vi "Transition State.vi"(8 "Error In":errorcluster, 10 "L       E \nIndicator":T1 caption="L      E", 11 "Present  State":T2) -> (0 "Error Out":errorcluster, 3 "Next State":T2)   [LabVIEW 2023]
doc: "This VI uses the present state and thre inputs L and E to determine the next state."
uses:
  controls/enum defining states.ctl
  controls/Boolean L E indictaor.ctl
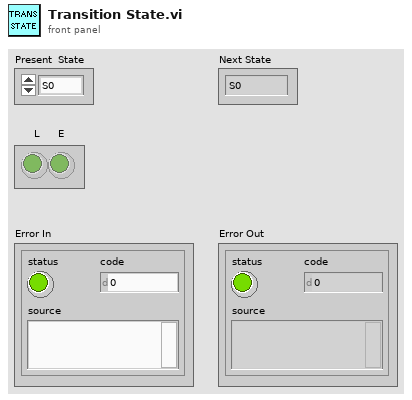
[diagram p1: front panel]
types:
  T1 = typedef "Boolean L E indictaor.ctl" = bool[]
  T2 = typedef "enum defining states.ctl" = enum16{"S0", "S1", "S2", "S3"}
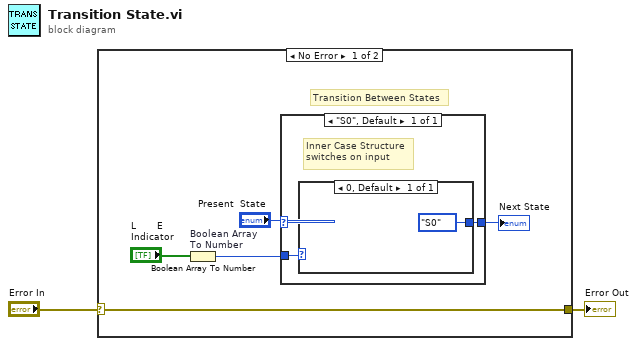
[diagram p0: block diagram]
diagram:
  n1 = case shown="No Error" "Error In" {
    selector: "Error In" -> [w6 w11]
    tunnel: [w6 w11] -> w1
    frame No Error {
      # "Transition Between States"
      n2 = Boolean Array To Number "Boolean Array\nTo Number"(Boolean array="L       E \nIndicator") -> (number=w5:u32)
      n3 = case shown="\"S0\", Default" "Present  State" {
        tunnel: [w9] -> w4
        tunnel: w5 -> [w8]
        frame "S0", Default {
          # "Inner Case Structure\nswitches on input"
          n4 = case shown="0, Default" w8 {
            tunnel: [enum_defining_states."S0" ("State Enum")] -> w9
            frame 0, Default {
            }
          }
        }
      }
      "Next State" <- w4
    }
    frame Error {
    }
  }
  "Error Out" <- w1
